vi "Waveform (G3) - Defaults.vi"() -> (0 "subcontrols":cluster{"persistent":T1, "sort":bool}, 1 "mask":bool[](array[boolean]), 2 "valid waveforms":T2[](array[typedef]), 3 "names":string[](array[string]))   [LabVIEW 2020, in "Waveform (G3).xctl"]
uses:
  Waveform (G3).xctl
  Waveform VIs/Waveform Enum (V3).ctl
  Noise (G3)/Noise (G3) - Persistent.ctl
  Noise (G3)/Noise (G3).xctl
panel:
  in  "Waveform":T2
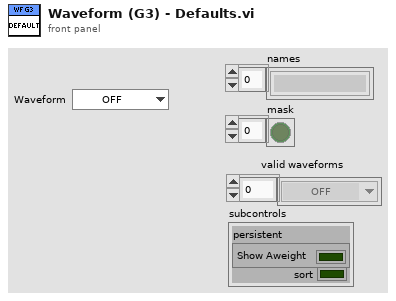
[diagram p1: front panel]
types:
  T1 = typedef "Noise (G3).xctl/Noise (G3) - Persistent.ctl" = cluster{"Show Aweight":bool}
  T2 = typedef "Waveform Enum (V3).ctl" = enum16{"OFF", "Tone", "Noise", "Pulse Train", "File", "FM Sweep", "Chirp Train", "Complex Tone", "FM Tone", "Vowel", "Ramp"}
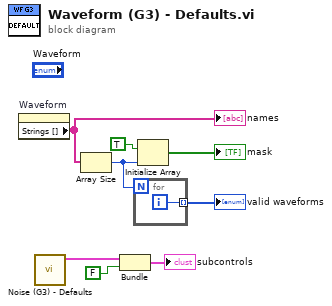
[diagram p0: block diagram]
diagram:
  n1 = property on="Waveform" class="Enum (strict)"() -> ("Strings []"=w7:string[])  [unwired: 2 in, 2 out]
  "names" <- w7
  n2 = call "Noise (G3) - Defaults.vi"() -> ("persistent"=w3:T1)  [unwired: 11 in]
  n3 = Array Size(array=w7) -> (size(s)=w4:i32)
  n4 = Bundle("persistent"=w3, FALSE) -> (→"subcontrols":cluster{"persistent":T1, bool})  [unwired: 1 in]
  n5 = for {
    N: w4 -> [_]
    tunnel: [w9] -> w5 mode=indexing
    i -> [w9]
  }
  "valid waveforms" <- w5
  n6 = Initialize Array(TRUE, w4) -> (→"mask":bool[])
